vi "Main.vi"() -> ()   [LabVIEW 2014]
uses:
  Enum.ctl
  Cacluator_class/Cacluator.lvclass
  Caculator.lvlib
panel:
  out "Result":dbl
  in  "a":dbl=1.0
  in  "b":dbl=2.0
  in  "Enum":T1
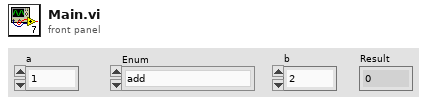
[diagram p1: front panel]
types:
  T1 = typedef "Caculator.lvlib/Enum.ctl" = enum16{"add", "subtract"}
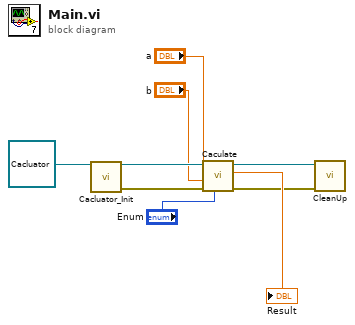
[diagram p0: block diagram]
diagram:
  n1 = call "Cacluator_Init.vi"("object in"=refnum<class "Cacluator.lvclass"> refnum ("Caculator.lvlib:Cacluator")) -> ("object out"=w8:refnum<class "Cacluator.lvclass">, "error out"=w7:errorcluster)  [unwired: 17 in]
  n2 = call "Caculate.vi"("Enum"="Enum", "error in (no error)"=w7, "b"="b", "a"="a", "Cacluator in"=w8) -> ("error out"=w1:errorcluster, "Result"=→"Result":dbl, "Cacluator out"=w2:refnum<class "Cacluator.lvclass">)  [unwired: 4 in]
  n3 = call-dynamic "CleanUp.vi"("object in"=w2, "error in (no error)"=w1) -> ()  [unwired: 16 in, 2 out]
